vi "C4Dev_startAcquisition.vi"(0 "c4dev in":refnum<k24>, 5 "nofBuf in":i64=4, 11 "error in (no error)":errorcluster) -> (4 "c4dev out":refnum<k24>, 15 "error out":errorcluster)   [LabVIEW 2015, in "libC4HdlLV.lvlib"]
uses:
  libC4HdlLV.lvlib
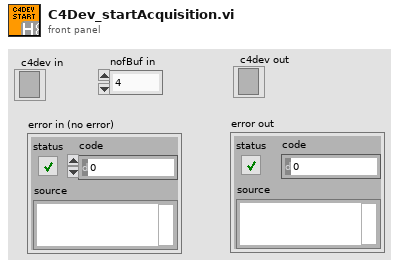
[diagram p1: front panel]
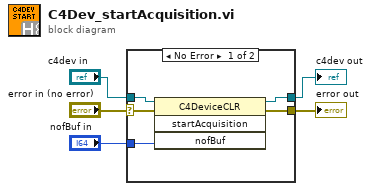
[diagram p0: block diagram]
diagram:
  n1 = case shown="No Error" "error in (no error)" {
    selector: "error in (no error)" -> [w6 w11]
    tunnel: "c4dev in" -> [w10 w12]
    tunnel: [w9 w12] -> w1
    tunnel: [w8 w11] -> w5
    tunnel: "nofBuf in" -> [w7 _]
    frame No Error {
      n2 = invoke class="C4DeviceCLR" method="startAcquisition"(reference=w10, error in=w6, "nofBuf"=w7) -> (reference out=w9:refnum<k24>, error out=w8:errorcluster)  [unwired: 1 in, 2 out]
    }
    frame Error {
    }
  }
  "error out" <- w5
  "c4dev out" <- w1
